vi "Variant_to_Enum_U16.vi"(8 "Error in":errorcluster, 11 "Value (in)":variant) -> (0 "Error out":errorcluster, 2 "Value (string)":string, 3 "Value (out)":u16(ring) items=["   128 x 128", "   256 x 128", "   256 x 256", "   512 x  64", "   512 x 128", "   512 x 256", "   512 x 512", "  1024 x 512", "  1024 x 1024", "   arbitrary"])   [LabVIEW 2012]
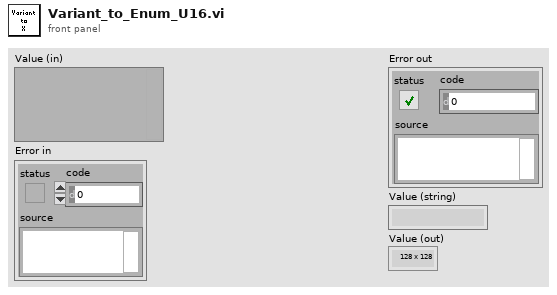
[diagram p1: front panel]
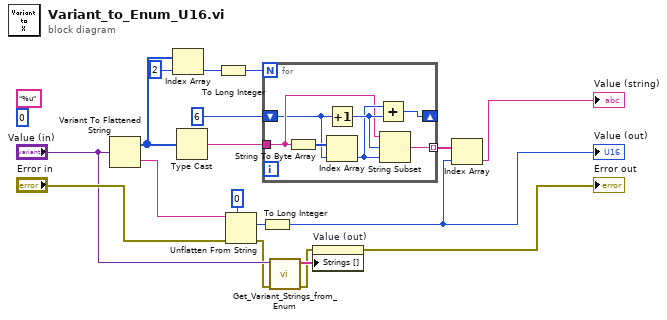
[diagram p0: block diagram]
diagram:
  (unwired) "%u" ("format string")
  (unwired) u16 0
  n1 = Variant To Flattened String(Variant="Value (in)") -> (data string=w13:string, 1:w17:i16[])
  n2 = Index Array(array=w17, index=2) -> (element=w8:i16)
  n3 = Type Cast(x=w17) -> (*(type *) &x=w14:string)  [unwired: 1 in]
  n4 = To Long Integer(number=w8) -> (32bit integer=w7:i32)
  n5 = Unflatten From String(type=u16 0, binary string=w13, error in (no error)="Error in") -> (value=w9:u16, error out=w3:errorcluster)  [unwired: 2 in, 1 out]
  n6 = To Long Integer(number=w9) -> (32bit integer=w6:i32)
  "Value (out)" <- w6
  n7 = for {
    N: w7 -> [_]
    tunnel: w14 -> [w22]
    shift-right: [w21] -> _
    shift-left: 6 ("index") -> [w19]
    tunnel: [w20] -> w16 mode=indexing
    n8 = String To Byte Array(string=w22) -> (unsigned byte array=w25:u8[])
    n9 = Increment(x=w19) -> (x+1=w24:i32)
    n10 = Index Array(array=w25, index=w19) -> (element=w23:u8)
    n11 = Add(x=w23, y=w24) -> (x+y=w21:i32)
    n12 = String Subset(string=w22, offset (0)=w24, length (rest)=w23) -> (substring=w20:string)
  }
  n13 = call "Get_Variant_Strings_from_Enum.vi"("error in (no error)"=w3, "Enum"="Value (in)") -> ("error out"=w1:errorcluster, "Enum strings"=w2:string[])  [unwired: 6 in, 2 out]
  n14 = property on="Value (out)" class="Ring (strict)"(error in=w1, "Strings []"=w2) -> (error out=→"Error out":errorcluster)  [unwired: 1 in, 1 out]
  n15 = Index Array(array=w16, index=w6) -> (element=→"Value (string)":string)
